vi "Create 2D Table.vi"(4 "use apostrophes (F)":bool, 8 "formatted values":string[][](array[string]), 11 "table name":string) -> (0 "can be indented?":bool, 3 "table":string)   [LabVIEW 2013, in "infolib.lvlib"]
uses:
  infolib.lvlib
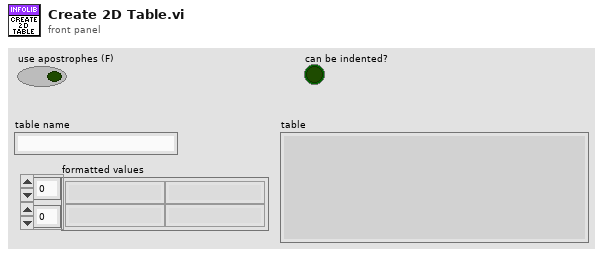
[diagram p1: front panel]
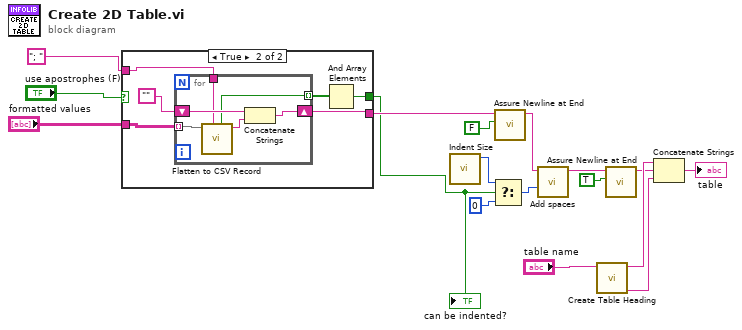
[diagram p0: block diagram]
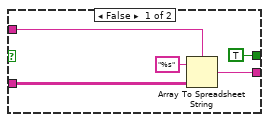
[diagram p2: hidden frame]
diagram:
  n1 = case shown="True" "use apostrophes (F)" {
    tunnel: [w21 w26] -> w8
    tunnel: "formatted values" -> [w20 w28]
    tunnel: "; " ("delimiter (Tab)") -> [w19 w25]
    tunnel: [TRUE w23] -> w2
    frame False {
      n2 = Array To Spreadsheet String(delimiter (Tab)=w19, array=w20, 3:"%s" ("format string")) -> (spreadsheet string=w21:string)
    }
    frame True {
      n3 = for {
        tunnel: w28 -> [w34] mode=indexing
        shift-right: [w31] -> w26
        shift-left: "" -> [w32]
        tunnel: w25 -> [w30]
        tunnel: [w29] -> w24 mode=indexing
        n4 = call "Flatten to CSV Record.vi"("delimiter (,)"=w30, "row of strings"=w34) -> ("CSV record"=w33:string, "can be indented?"=w29:bool)  [unwired: 7 in, 1 out]
        n5 = Concatenate Strings(w32, w33) -> (w31:string)
      }
      n6 = And Array Elements(Boolean array=w24) -> (logical AND=w23:bool)
    }
  }
  "can be indented?" <- w2
  n7 = call "Indent Size.vi"() -> ("indent size"=w3:i32)  [unwired: 10 in, 1 out]
  n8 = Select(t=w3, s=w2, f=0) -> (s? t:f=w4:i32)
  n9 = call "Assure Newline at End.vi"("Set End Of Line (F)"=FALSE, "string"=w8) -> ("string out"=w12:string)  [unwired: 9 in]
  n10 = call "Add spaces.vi"("spaces no"=w4, "input string"=w12) -> ("result string"=w10:string)  [unwired: 9 in]
  n11 = call "Create Table Heading.vi"("table name"="table name") -> ("table end"=w15:string, "table start"=w16:string)  [unwired: 9 in]
  n12 = call "Assure Newline at End.vi"("Set End Of Line (F)"=TRUE, "string"=w10) -> ("string out"=w9:string)  [unwired: 9 in]
  n13 = Concatenate Strings(w16, w9, w15) -> (→"table":string)
